vi "LVClass_CameraSet Reset to factory parameters.vi"(0 "CameraSet.lvclass":refnum<class "CameraSet.lvclass">, 11 "error in (no error)":errorcluster) -> (4 "CameraSet.lvclass":refnum<class "CameraSet.lvclass">, 15 "error out":errorcluster)   [LabVIEW 2020, in "CameraSet.lvclass"]
doc: "Reset parameters to factory values (default values). see also the LVClass_CameraSet Reset CameraParameter to DefaultValue.vi method to reset to default values with more options\n\n<B>CameraSetIn</B> : Camera object.\n<B>CameraSetOut</B> : Camera object."
uses:
  CameraSet.lvclass
  CameraSet.lvclass/CameraSet.ctl
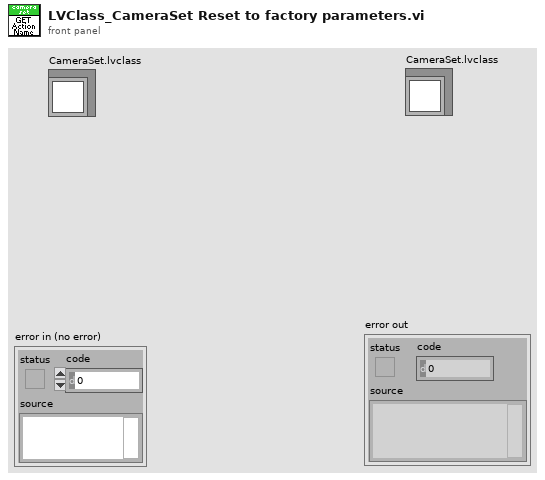
[diagram p1: front panel]
types:
  T1 = typedef "ClassID.ctl" = i64
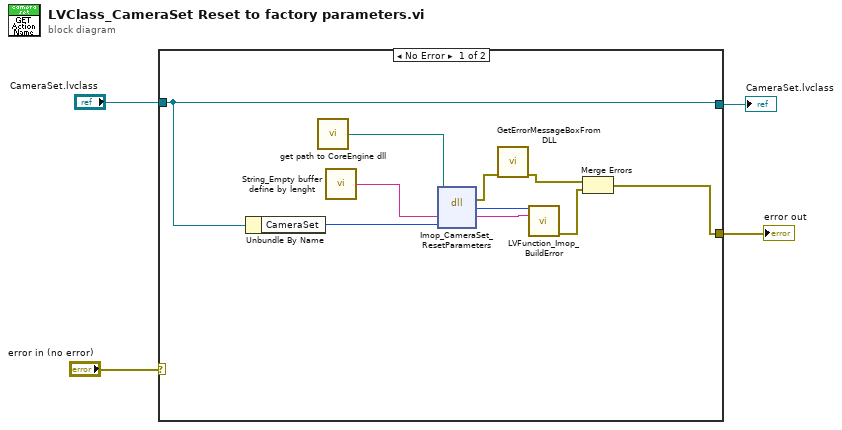
[diagram p0: block diagram]
diagram:
  n1 = case shown="No Error" "error in (no error)" {
    selector: "error in (no error)" -> [_ w15]
    tunnel: "CameraSet.lvclass" -> [w9 w16]
    tunnel: [w9 w16] -> w2
    tunnel: [w5 w15] -> w1
    frame No Error {
      n2 = Unbundle By Name(w9) -> ("CameraSet"=w8:T1)
      n3 = call "get path to CoreEngine dll.vi"() -> ("path to wavekit library"=w11:path)  [unwired: 14 in, 1 out]
      n4 = call "String_Empty buffer define by lenght.vi"() -> ("Empty buffer"=w12:string)  [unwired: 1 in]
      n5 = dll-call lib="D:/soft/HASO_v3/SVN_trunk/ImOpCoreEngine4_LV2011/DLLs/c_interface_vc100.dll" fn="Imop_CameraSet_ResetParameters"(path in=w11, "message"=w12, "objet"=w8) -> (error out=w10:errorcluster, "return type"=w14:i32, "message"=w13:string)  [unwired: 3 in, 1 out]
      n6 = call "GetErrorMessageBoxFromDLL.vi"("error IN"=w10) -> ("error OUT"=w7:errorcluster)  [unwired: 10 in]
      n7 = call "LVFunction_Imop_BuildError.vi"("code"=w14, "String to Prepend to source (\"\")"=w13) -> ("error out"=w6:errorcluster)  [unwired: 13 in]
      n8 = Merge Errors(w7, w6) -> (w5:errorcluster)
    }
    frame Error {
    }
  }
  "CameraSet.lvclass" <- w2
  "error out" <- w1
